vi "MultiD Array to JSON.vi"(7 "Treatment of Infinity/NaN":T1, 8 "error in (no error)":errorcluster, 10 "Array Dimensions":i32[](array[numeric]), 11 "Variant Data":T2[](array[typedef])) -> (0 "error out":errorcluster, 2 "JSON Array out":refnum<class "JSON Array.lvclass">, 3 "Remaining Variant Data":T2[](array[typedef]))   [LabVIEW 2011, in "Variant JSON.lvlib"]
uses:
  Variant JSON.lvlib
  JSON Scalar/variants/Variant Data Typdef.ctl
  <vilib>/Utility/VariantDataType/Type.ctl
  JSON Array/JSON Array.lvclass
  JSON Scalar/Infinity&NaN.ctl
  JSON Value/JSON Value.lvclass
  <vilib>/Utility/VariantDataType/VariantType.lvlib
  JSON Scalar/JSON Scalar.lvclass
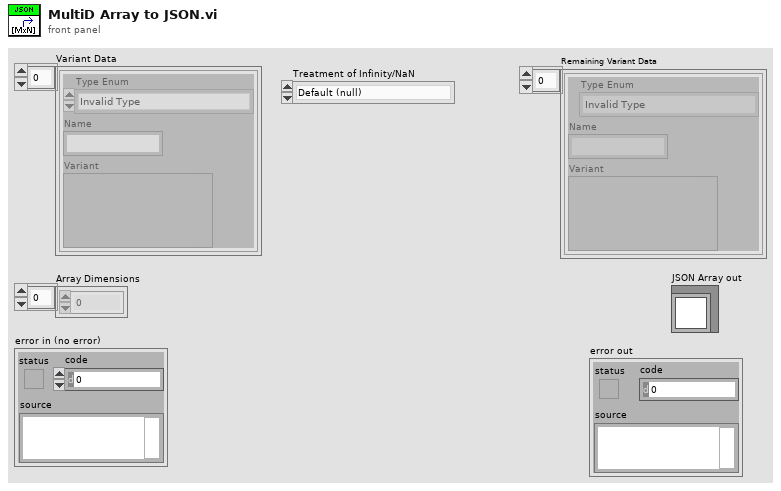
[diagram p1: front panel]
types:
  T1 = typedef "JSON Scalar.lvclass/Infinity&NaN.ctl" = enum16{"Default (null)", "Extended", "LabVIEW extensions"}
  T2 = typedef "JSON Scalar.lvclass/Variant Data Typdef.ctl" = cluster{"Type Enum":T3, "Name":string, "Variant":variant}
  T3 = typedef "VariantType.lvlib/Type.ctl" = enum8{"Invalid Type", "Void", "I8", "I16", "I32", "I64", "U8", "U16", "U32", "U64", "Single Float", "Double Float", "Extended Float", "Single Complex", "Double Complex", "Extended Complex", "Enum U8", "Enum U16", "Enum U32", "Enum U64", "Single Float With Unit", "Double Float With Unit", "Extended Float With Unit", "Single Complex with Unit", "Double Complex with Unit", "Extended Complex with Unit", "Boolean", "String", "Path", "Picture", "Tag", "Array", "Cluster", "Variant", "LV Variant", "Waveform", "Timestamp", "Digital Waveform", "Digital Data", "ExpressData", "Refnum", "External Data", "VI", "Poly VI", "LabVIEW Class Instance", "Fixed Point"}
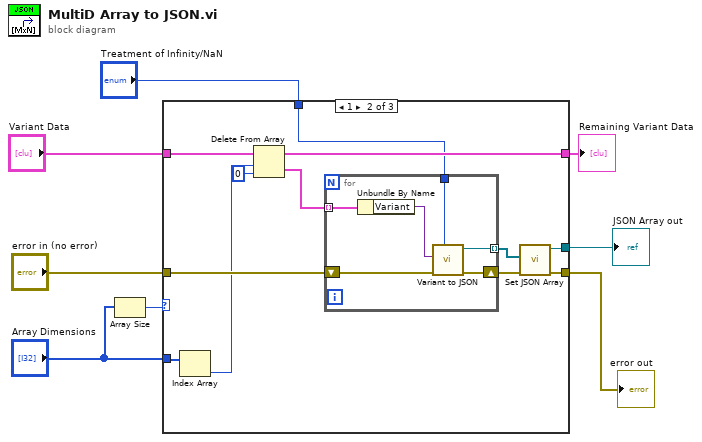
[diagram p0: block diagram]
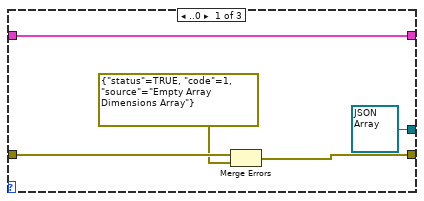
[diagram p2: hidden frame]
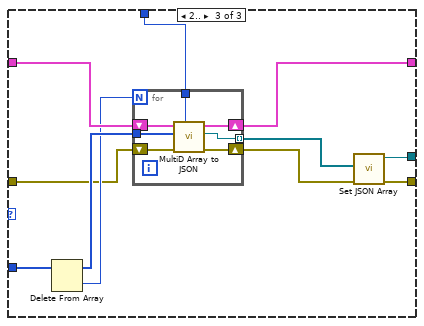
[diagram p3: hidden frame]
diagram:
  n1 = Array Size(array="Array Dimensions") -> (size(s)=w4:i32)
  n2 = case shown="1" w4 {
    tunnel: "Variant Data" -> [w11 w19 w41]
    tunnel: "error in (no error)" -> [w13 w25 w34]
    tunnel: [w10 w24 w35] -> w6
    tunnel: [refnum<class "JSON Array.lvclass"> refnum ("JSON Array out") w21 w36] -> w5
    tunnel: "Array Dimensions" -> [_ w20 w42]
    tunnel: [w11 w16 w40] -> w2
    tunnel: "Treatment of Infinity/NaN" -> [_ w14 w32]
    frame ..0 {
      n3 = Merge Errors(w13, errorcluster {"status"=TRUE, "code"=1, "source"="Empty Array Dimensions Array"} ("error in")) -> (w10:errorcluster)
    }
    frame 1 {
      n4 = Index Array(array=w20) -> (element=w18:i32)  [unwired: 1 in]
      n5 = Delete From Array(array=w19, length=w18, index=0) -> (deleted portion=w17:T2[], array with subset deleted=w16:T2[])
      n6 = for {
        tunnel: w17 -> [w31] mode=indexing
        tunnel: [w30] -> w22 mode=indexing
        shift-right: [w28] -> w23
        shift-left: w25 -> [w29]
        tunnel: w14 -> [w26]
        n7 = Unbundle By Name(w31) -> ("Variant"=w27:variant)
        n8 = call "Variant to JSON.vi"("Treatment of Infinity/NaN"=w26, "error in (no error)"=w29, "Variant"=w27) -> ("error out"=w28:errorcluster, "JSON Value out"=w30:refnum<class "JSON Value.lvclass">)  [unwired: 7 in]
      }
      n9 = call "Set JSON Array.vi"("error in (no error)"=w23, "Array"=w22) -> ("error out"=w24:errorcluster, "JSON Array out"=w21:refnum<class "JSON Array.lvclass">)  [unwired: 8 in]
    }
    frame 2.. {
      n10 = Delete From Array(array=w42) -> (deleted portion=w38:i32, array with subset deleted=w39:i32[])  [unwired: 2 in]
      n11 = for {
        N: w38 -> [_]
        tunnel: w39 -> [w47]
        tunnel: [w46] -> w37 mode=indexing
        shift-right: [w44] -> w33
        shift-left: w34 -> [w45]
        shift-right: [w48] -> w40
        shift-left: w41 -> [w49]
        tunnel: w32 -> [w43]
        n12 = call "MultiD Array to JSON.vi"("Treatment of Infinity/NaN"=w43, "error in (no error)"=w45, "Array Dimensions"=w47, "Variant Data"=w49) -> ("error out"=w44:errorcluster, "JSON Array out"=w46:refnum<class "JSON Array.lvclass">, "Remaining Variant Data"=w48:T2[])  [unwired: 5 in]
      }
      n13 = call "Set JSON Array.vi"("error in (no error)"=w33, "Array"=w37) -> ("error out"=w35:errorcluster, "JSON Array out"=w36:refnum<class "JSON Array.lvclass">)  [unwired: 8 in]
    }
  }
  "error out" <- w6
  "JSON Array out" <- w5
  "Remaining Variant Data" <- w2
